vi "Windspeed Warnings.vi"(10 "Max Windspeed":dbl, 11 "Current Windspeed":dbl) -> (2 "Windspeed Warning Text":string="No Warning", 3 "Windspeed Warning?":bool)   [LabVIEW 2012]
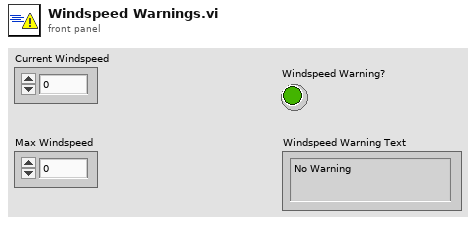
[diagram p1: front panel]
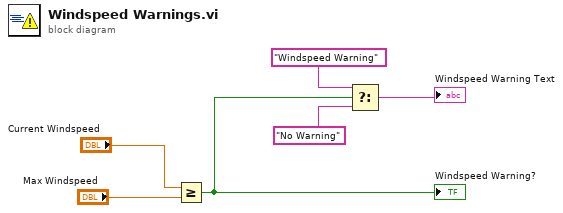
[diagram p0: block diagram]
diagram:
  n1 = Greater Or Equal?(x="Current Windspeed", y="Max Windspeed") -> (x >= y?=w4:bool)
  "Windspeed Warning?" <- w4
  n2 = Select(t="Windspeed Warning", s=w4, f="No Warning") -> (s? t:f=→"Windspeed Warning Text":string)
